vi "SPVM parser.vi"(8 "error in (no error)":errorcluster, 9 "Sample data":bool, 10 "Render graph":bool, 11 "3D Plot lvclass Array in":refnum<class "3D Plot Datatype.lvclass">[](array[class])) -> (0 "error out":errorcluster, 3 "3D Plot lvclass Array out":refnum<class "3D Plot Datatype.lvclass">[](array[class]))   [LabVIEW 2020]
uses:
  <vilib>/Math Plots/3D Math Plots/3D Plot/3D Plot Datatype/3D Plot Datatype.lvclass
  <vilib>/Math Plots/3D Math Plots/3D Scatter/3D Scatter XCtrl/3D Scatter.xctl
  <vilib>/Utility/file.llb/Read Delimited Spreadsheet (DBL).vi
  <vilib>/Math Plots/3D Math Plots/3D Scatter/3D Scatter Datatype/Public/Plot Helper (Vector).vi
  <vilib>/Math Plots/3D Math Plots/3D Scatter/3D Scatter Datatype/3D Scatter Datatype.lvclass
panel:
  out "3D Scatter 2":refnum<class "3D Plot Datatype.lvclass">[](xcontrol)
  in  "File settings":T1={"Scale ( um )"=50, "Morphology"="Hexagonal unit cell, rhombohedral bravais lattice", "Raster"="Spiral"}
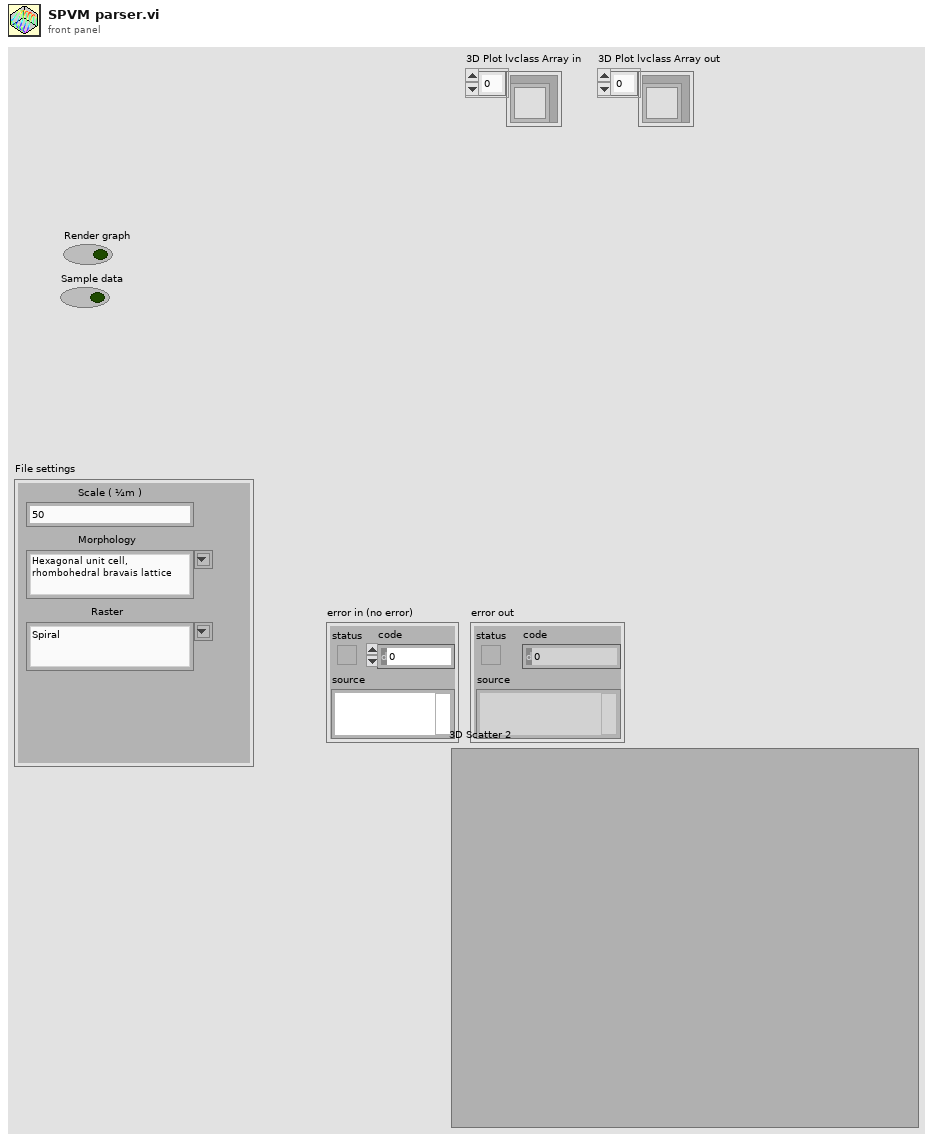
[diagram p1: front panel]
types:
  T1 = cluster{"Scale ( um )":i16, "Morphology":string, "Raster":string}
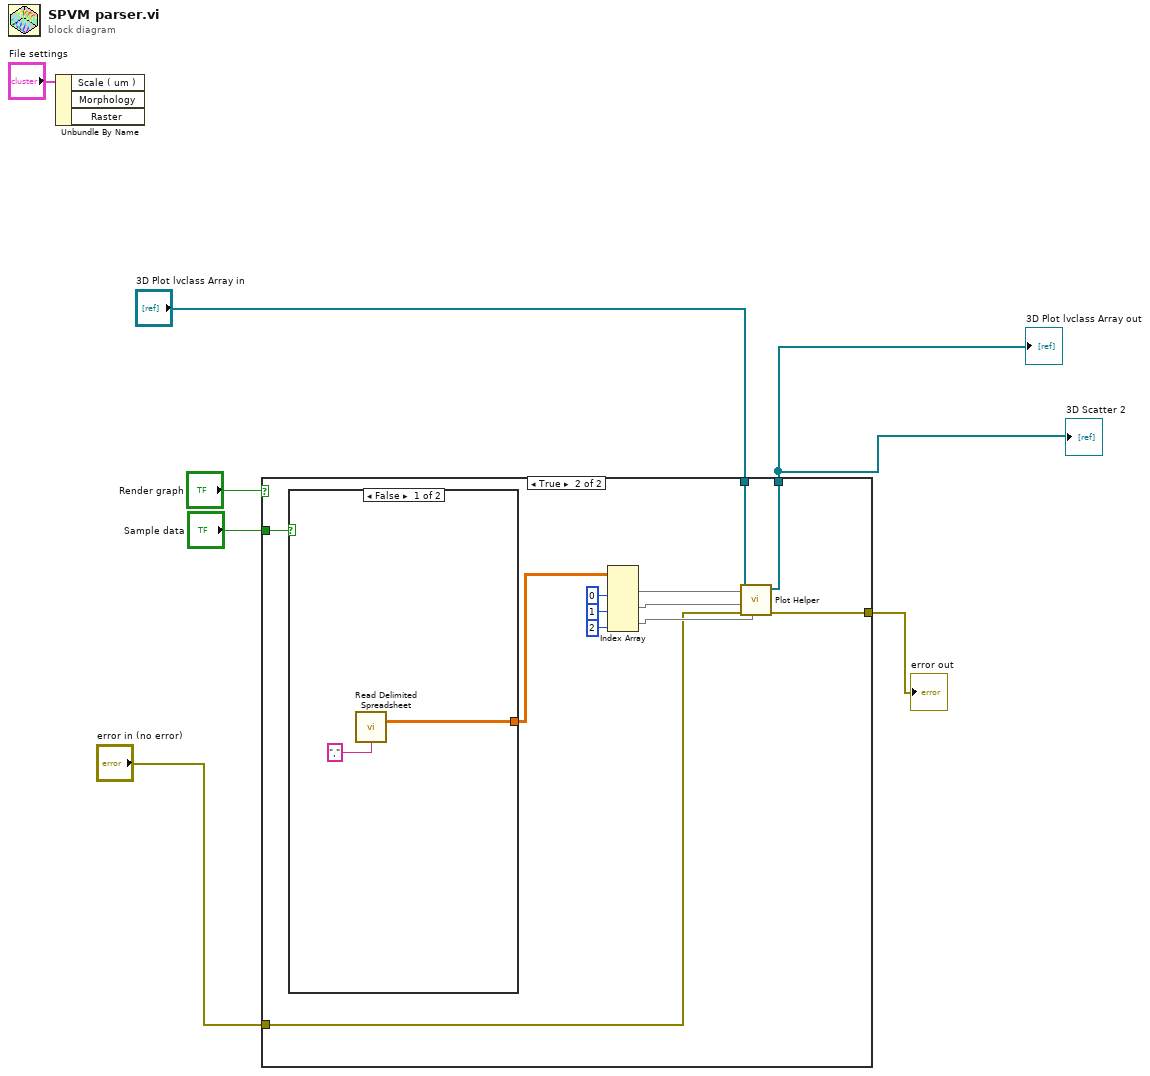
[diagram p0: block diagram]
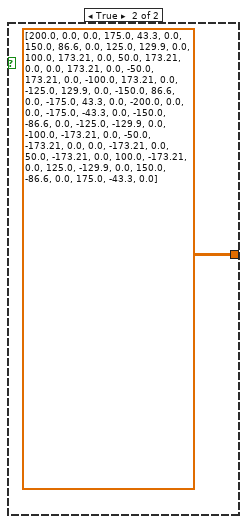
[diagram p3: hidden frame]
diagram:
  n1 = Unbundle By Name("File settings") -> ()  [unwired: 3 out]
  n2 = case shown="True" "Render graph" {
    tunnel: "Sample data" -> [_ w21]
    tunnel: "error in (no error)" -> [w8 w17]
    tunnel: "3D Plot lvclass Array in" -> [w9 w16]
    tunnel: [w8 w12] -> w2
    tunnel: [w9 w11] -> w1
    frame False {
    }
    frame True {
      n3 = case shown="False" w21 {
        tunnel: [w23 dbl[][] [[200.0, 0.0, 0.0], [175.0, 43.3, 0.0], [150.0, 86.6, 0.0], [125.0, 129.9, 0.0], [100.0, 173.21, 0.0], [50.0, 173.21, 0.0], [0.0, 173.21, 0.0], [-50.0, 173.21, 0.0], [-100.0, 173.21, 0.0], [-125.0, 129.9, 0.0], [-150.0, 86.6, 0.0], [-175.0, 43.3, 0.0], [-200.0, 0.0, 0.0], [-175.0, -43.3, 0.0], [-150.0, -86.6, 0.0], [-125.0, -129.9, 0.0], [-100.0, -173.21, 0.0], [-50.0, -173.21, 0.0], [0.0, -173.21, 0.0], [50.0, -173.21, 0.0], [100.0, -173.21, 0.0], [125.0, -129.9, 0.0], [150.0, -86.6, 0.0], [175.0, -43.3, 0.0]] ("all rows")] -> w10
        frame False {
          n4 = call-poly <vilib>:"Read Delimited Spreadsheet.vi"("delimiter (\\t)"="," ("delimiter (\\t)")) -> ("all rows"=w23:dbl[][])  [unwired: 9 in, 5 out]
        }
        frame True {
        }
      }
      n5 = Index Array(array=w10, index (col) #1=0 ("disabled index (col)"), index (col) #2=1 ("index (col)"), index (col) #3=2 ("index (col)")) -> (element #1=w18:dbl[], element #2=w19:dbl[], element #3=w20:dbl[])  [unwired: 3 in]
      n6 = call-poly <vilib>:"Plot Helper.vi"("z vector"=w20, "error in (no error)"=w17, "y vector"=w19, "x vector"=w18, "3D Plot lvclass Array in"=w16) -> ("error out"=w12:errorcluster, "3D Plot lvclass Array out"=w11:refnum<class "3D Plot Datatype.lvclass">[])  [unwired: 1 in, 4 out]
    }
  }
  "3D Plot lvclass Array out" <- w1
  "error out" <- w2
  "3D Scatter 2" <- w1
